vi "FunGobel_USBGEA.vi"(7 "Enum":enum16{"Read", "Write"}(ring), 8 "error in":errorcluster, 11 "GEA2 RefIN":refnum<k24>) -> (0 "error out":errorcluster, 2 ".not. x?":bool, 3 "GEA2 RefOut":refnum<k24>)   [LabVIEW 2013]
uses:
  C:/Automation/DLLS/PC Tools .NET/GeaCommunication.dll
  Automation/DLLS/PC Tools .NET/GeaCommunication.dll
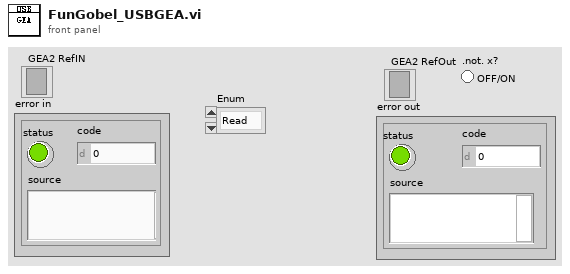
[diagram p1: front panel]
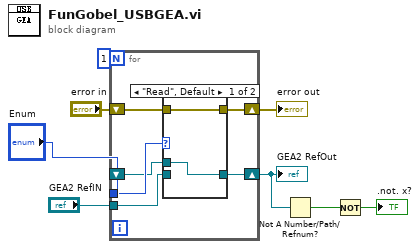
[diagram p0: block diagram]
diagram:
  n1 = for {
    N: 1 -> [_]
    tunnel: "Enum" -> [w14]
    shift-right: [w13] -> w4
    shift-left: _ -> [w12]
    shift-right: [w11] -> w7
    shift-left: "error in" -> [w10]
    tunnel: "GEA2 RefIN" -> [w9]
    n2 = case shown="\"Read\", Default" w14 {
      tunnel: [w16 w18] -> w13
      tunnel: w12 -> [w16 _]
      tunnel: [w15 w17] -> w11
      tunnel: w10 -> [w15 w17]
      tunnel: w9 -> [_ w18]
      frame "Read", Default {
      }
      frame "Write" {
      }
    }
  }
  "GEA2 RefOut" <- w4
  "error out" <- w7
  n3 = Not A Number/Path/Refnum?(number/path/refnum=w4) -> (NaN/Path/Refnum?=w3:bool)
  n4 = Not(x=w3) -> (.not. x?=→".not. x?":bool)
